vi "Start! globals.vi"() -> ()   [LabVIEW 2011]
panel:
  in  "VIs to Run":T1(array[cluster])=[{"VI name"="Glimpse Launcher.vi", "Location"=enum."Glimpse", "Run"=TRUE, "Minimized?"=TRUE, "Subdirectory (w trailing \"\\\")"=""}, {"VI name"="shutters activate.vi", "Location"=enum."Plug-ins", "Run"=TRUE, "Minimized?"=FALSE, "Subdirectory (w trailing \"\\\")"="newhnu shutters\\"}, {"VI name"="Multi-mode acquisition.vi", "Location"=enum."Plug-ins", "Run"=TRUE, "Minimized?"=FALSE, "Subdirectory (w trailing \"\\\")"=""}, {"VI name"="RR autofocus view-calibrate.vi", "Location"=enum."Plug-ins", "Run"=TRUE, "Minimized?"=FALSE, "Subdirectory (w trailing \"\\\")"=""}, {"VI name"="Camera startup.vi", "Location"=enum."Plug-ins", "Run"=TRUE, "Minimized?"=FALSE, "Subdirectory (w trailing \"\\\")"="Camera\\"}, {"VI name"="stage controller.vi", "Location"=enum."Plug-ins", "Run"=TRUE, "Minimized?"=FALSE, "Subdirectory (w trailing \"\\\")"="Stage\\"}, {"VI name"="knob driver 3.vi", "Location"=enum."Plug-ins", "Run"=TRUE, "Minimized?"=TRUE, "Subdirectory (w trailing \"\\\")"="phidgets knobs\\"}, {"VI name"="Autofocus Globals.vi", "Location"=enum."Plug-ins", "Run"=FALSE, "Minimized?"=FALSE, "Subdirectory (w trailing \"\\\")"=""}, {"VI name"="GPI-Load-Save settings.vi", "Location"=enum."Glimpse", "Run"=TRUE, "Minimized?"=FALSE, "Subdirectory (w trailing \"\\\")"=""}, {"VI name"="RR asynchronous autofocus.vi", "Location"=enum."Plug-ins", "Run"=FALSE, "Minimized?"=FALSE, "Subdirectory (w trailing \"\\\")"=""}, {"VI name"="Ixon z-stack acquisition.vi", "Location"=enum."Plug-ins", "Run"=FALSE, "Minimized?"=TRUE, "Subdirectory (w trailing \"\\\")"="ixon camera\\"}]
  in  "Plug-ins folder or .llb file":path=path "C:/Users/gelles/Documents/GitHub/Glimpse/Microscope plugins"
  in  "Glimpse folder or .llb":path=path "C:/Users/gelles/Documents/GitHub/Glimpse/Glimpse core"
  # "Note:  If this VI is inside an LLB, the above folder names are ignored and the \nLLB name is used instead"
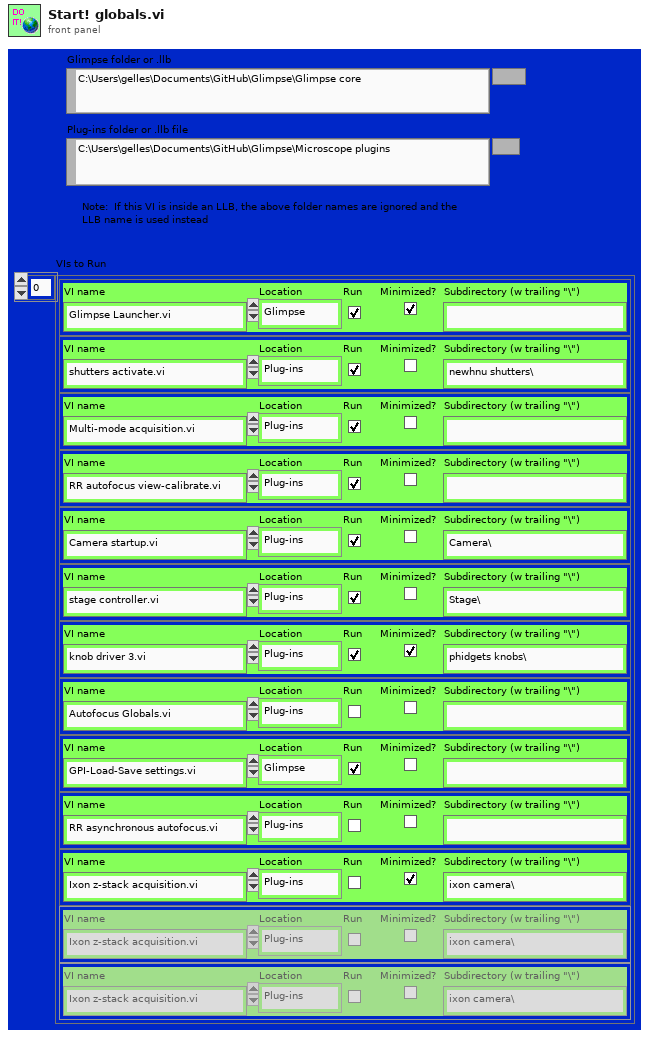
[diagram p1: front panel]
types:
  T1 = cluster{"VI name":string, "Location":enum16{"Plug-ins", "Glimpse"}, "Run":bool, "Minimized?":bool, "Subdirectory (w trailing \"\\\")":string}[]
diagram:
